vi "water tank.vi"() -> ()   [LabVIEW 2024]
panel:
  out "Warning txt":string
  in  "MAx level":dbl
  in  "Min level":dbl
  in  "Setpoint":dbl
  out "Tank":dbl(slide) scale=0.0..100.0
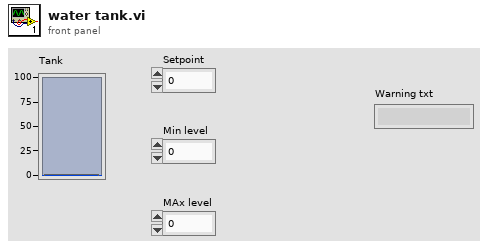
[diagram p1: front panel]
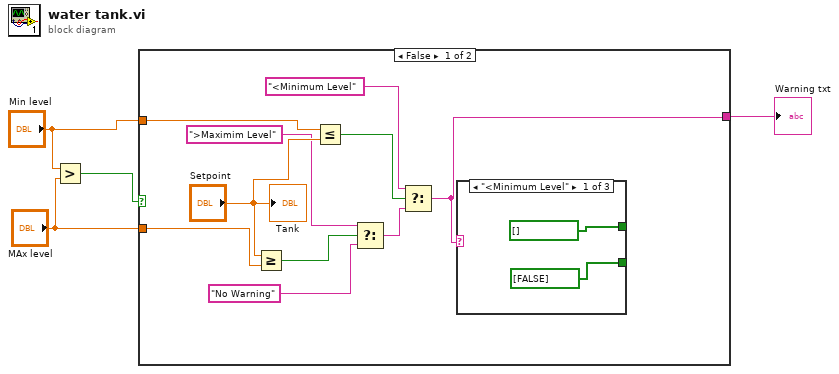
[diagram p0: block diagram]
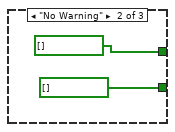
[diagram p2: hidden frame]
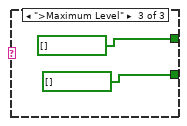
[diagram p3: hidden frame]
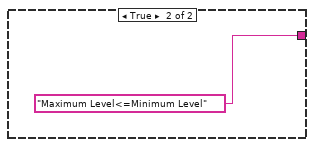
[diagram p4: hidden frame]
diagram:
  n1 = Greater?(x="Min level", y="MAx level") -> (0:w1:bool)
  n2 = case shown="False" w1 {
    tunnel: "MAx level" -> [w14 _]
    tunnel: "Min level" -> [w12 _]
    tunnel: [w5 "Maximum Level<=Minimum Level"] -> w2
    frame False {
      n3 = Greater Or Equal?(x="Setpoint", y=w14) -> (x >= y?=w8:bool)
      n4 = Less Or Equal?(x=w12, y="Setpoint") -> (x <= y?=w11:bool)
      n5 = Select(t=">Maximim Level", s=w8, f="No Warning") -> (s? t:f=w6:string)
      n6 = Select(t="<Minimum Level", s=w11, f=w6) -> (s? t:f=w5:string)
      n7 = case shown="\"<Minimum Level\"" w5 {
        tunnel: [bool[] [] bool[] [] bool[] []] -> _
        tunnel: [bool[] [FALSE] bool[] [] bool[] []] -> _
        frame "<Minimum Level" {
        }
        frame "No Warning" {
        }
        frame ">Maximum Level" {
        }
      }
      "Tank" <- "Setpoint"
    }
    frame True {
    }
  }
  "Warning txt" <- w2
